vi "UartIOSet.vi"(8 "error in (no error)":errorcluster caption="错误输入（无错误）", 9 "RX IO(0~15)":i32=1, 10 "TX IO(0~15)":i32, 11 "handle":u64) -> (0 "error out":errorcluster caption="错误输出", 2 "function return":i32, 3 "handle out":u64)   [LabVIEW 2018]
doc: "Set pos. or neg. Supply voltage"
uses:
  InstrumentsPlayground.lvlib
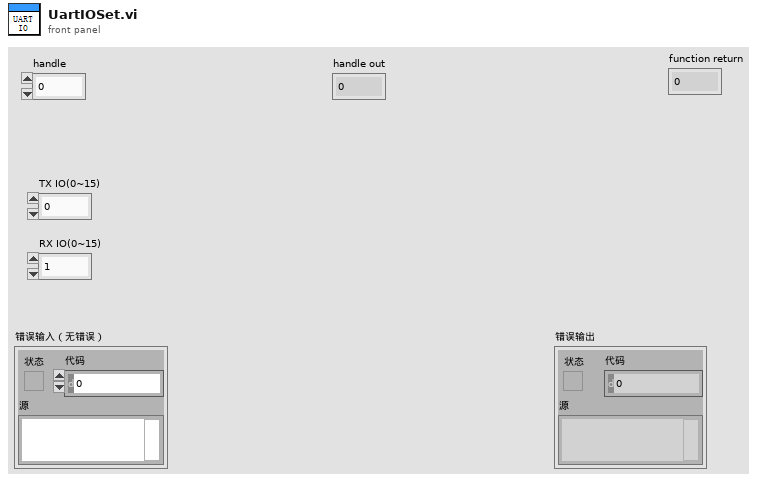
[diagram p1: front panel]
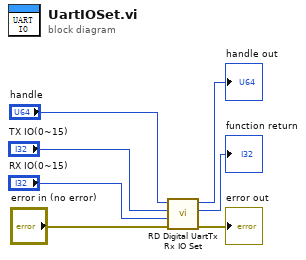
[diagram p0: block diagram]
diagram:
  n1 = call "RD Digital UartTx Rx IO Set.vi"("error in (no error)"="error in (no error)", "RxDIO"="RX IO(0~15)", "TxDIO"="TX IO(0~15)", "handle"="handle") -> ("error out"=→"error out":errorcluster, "function return"=→"function return":i32, "handle out"=→"handle out":u64)  [unwired: 5 in]
